vi "CreateScanPattern_LS1.vi"(8 "Error in":errorcluster, 11 "VarParam":string caption="Paramètre de balayage:") -> (0 "Error out":errorcluster, 1 "ModèleSauv":i32, 2 "SavedOK":bool, 3 "Modèles out":string[](array[string]))   [LabVIEW 2010]
doc: "Ce Vi sert à la création de modèles de balayages. À partir des positions de départ, de fin et du pas du balayage, il crée une liste de position qui constitue le modèle. Le VI permet ensuite la sauvegarde des nouveaux modèles et la gestion des modèles existant."
uses:
  <vilib>/Utility/error.llb/DialogType.ctl
  <vilib>/Utility/config.llb/NI_LVConfig.lvlib
panel:
  out "VarParamOut":string caption="Paramètre de balayage:"
  in  "InclFin":bool=TRUE caption="Inclure la \nposition finale"
  in  "Positions":dbl[](array[numeric])=[-100.0, -90.0, -80.0, -70.0, -60.0, -50.0, -40.0, -30.0, -20.0, -10.0, 0.0, 10.0, 20.0, 30.0, 40.0, 50.0, 60.0, 70.0, 80.0, 90.0, 100.0, 110.0, 120.0, 130.0, 140.0, 150.0, 160.0, 170.0, 180.0, 190.0, 200.0, 210.0, 220.0, 230.0, 240.0, 250.0, 260.0, 270.0, 280.0, 290.0, 300.0, 310.0, 320.0, 330.0, 340.0, 350.0, 360.0, 370.0, 380.0, 390.0, 400.0, 410.0, 420.0, 430.0, 440.0, 450.0, 460.0, 470.0, 480.0, 490.0, 500.0, 510.0, 520.0, 530.0, 540.0, 550.0, 560.0, 570.0, 580.0, 590.0, 600.0, 610.0, 620.0, 630.0, 640.0, 650.0, 660.0, 670.0, 680.0, 690.0, 700.0, 710.0, 720.0, 730.0, 740.0, 750.0, 760.0, 770.0, 780.0, 790.0, 800.0, 810.0, 820.0, 830.0, 840.0, 850.0, 860.0, 870.0, 880.0, 890.0, 900.0, 910.0, 920.0, 930.0, 940.0, 950.0, 960.0, 970.0, 980.0, 990.0, 1000.0] min=-2.0 max=770.0 step=0.01 format="%.2f"
  in  "OK":bool
  in  "Save":bool
  in  "Ajouter":bool
  in  "Effacer":bool
  in  "Fin":dbl=770.0 format="%.2f"
  in  "Pas":dbl=0.1 format="%.2f"
  in  "Départ":dbl=770.0 format="%.2f"
  in  "Nom du modèle":string
  in  "Modèles":i32(listbox) caption="Modèles de Balayage"
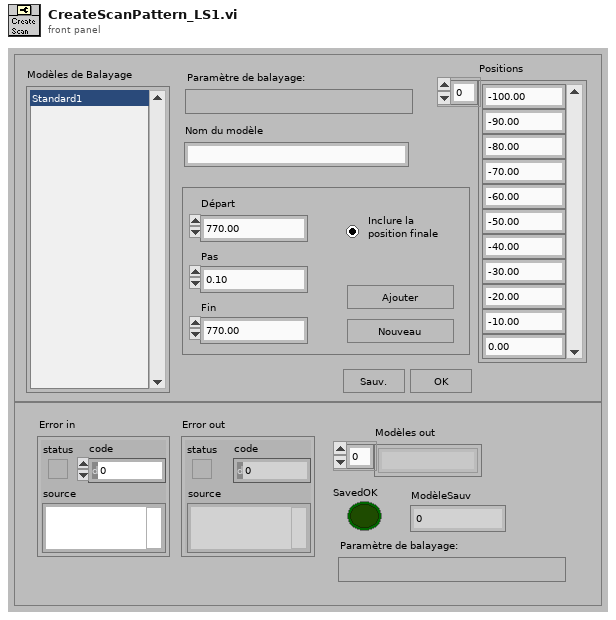
[diagram p1: front panel]
types:
  T1 = typedef "DialogType.ctl" = u16
  T2 = typedef "NI_LVConfig.lvlib/Config Data RefNum.ctl" = refnum<k1>
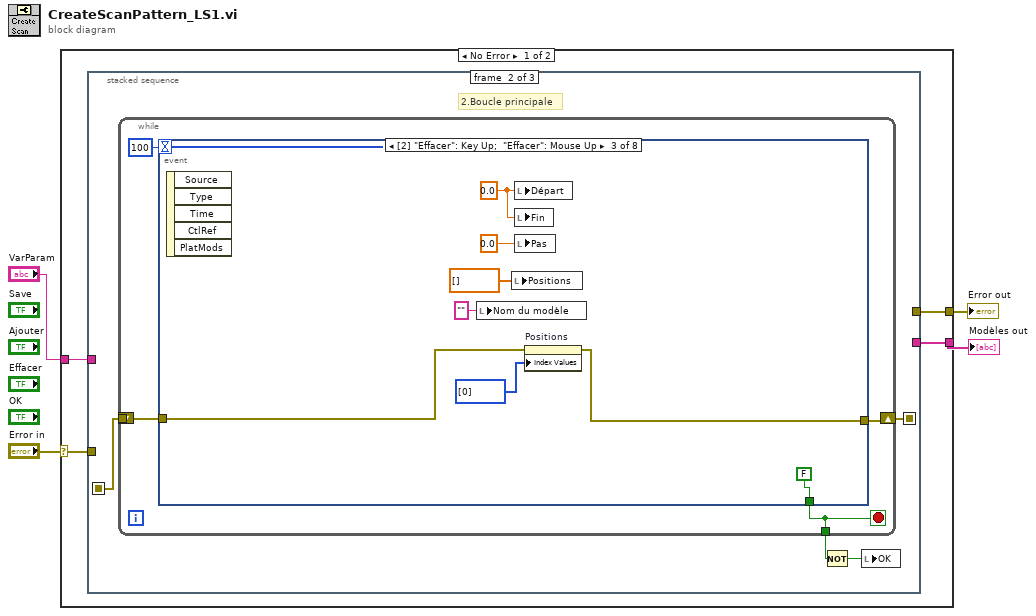
[diagram p0: block diagram]
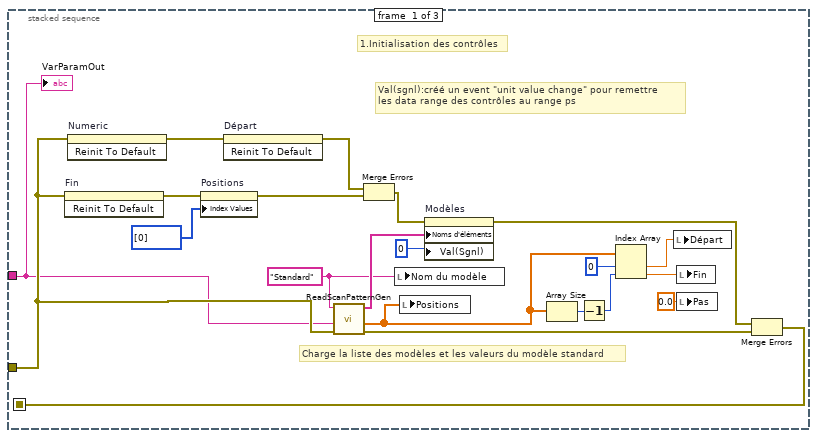
[diagram p2: hidden frame]
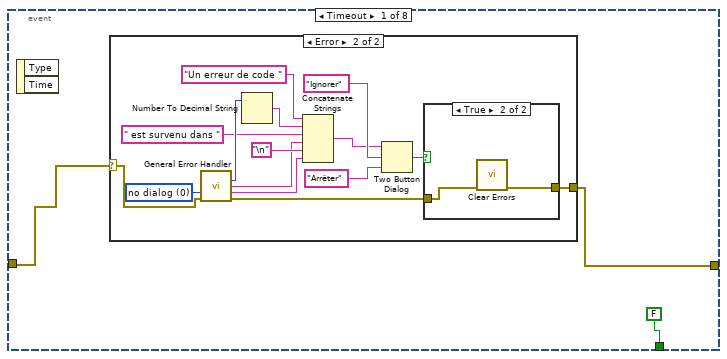
[diagram p3: hidden frame]
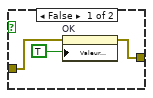
[diagram p5: hidden frame]
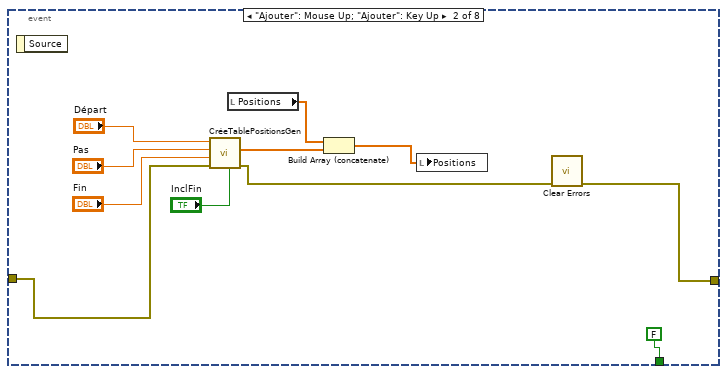
[diagram p6: hidden frame]
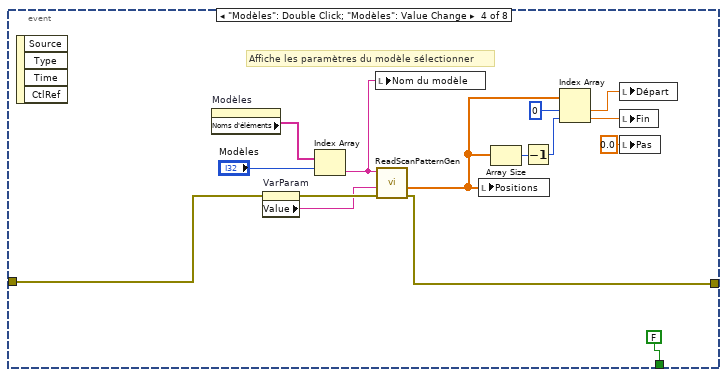
[diagram p7: hidden frame]
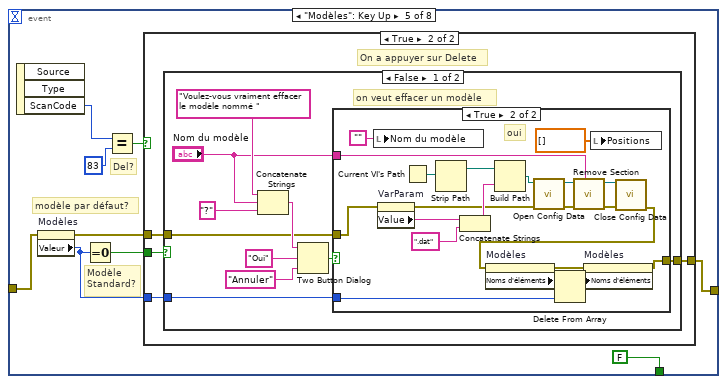
[diagram p8: hidden frame]
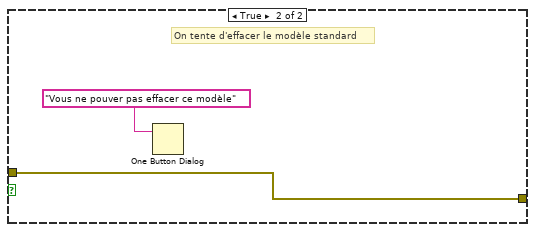
[diagram p11: hidden frame]
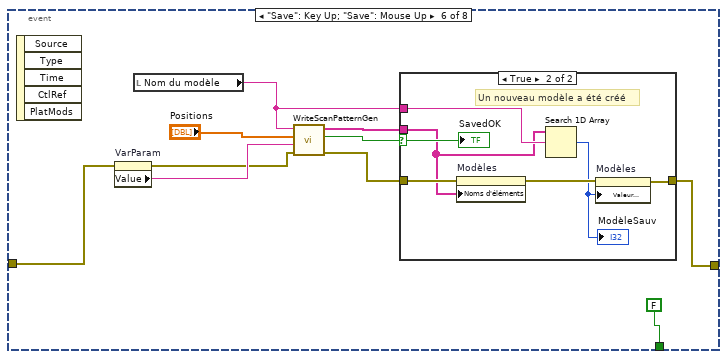
[diagram p12: hidden frame]
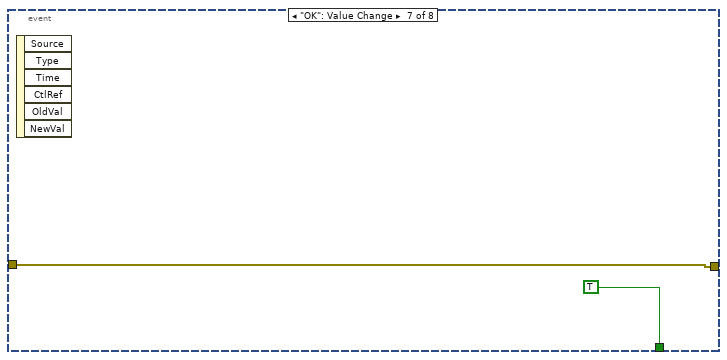
[diagram p14: hidden frame]
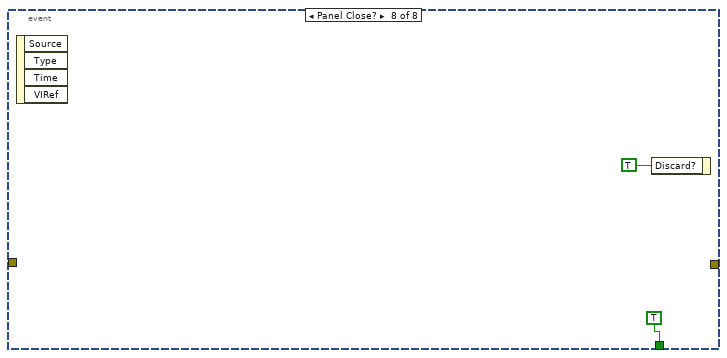
[diagram p15: hidden frame]
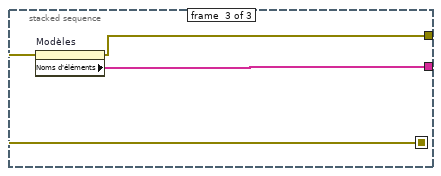
[diagram p16: hidden frame]
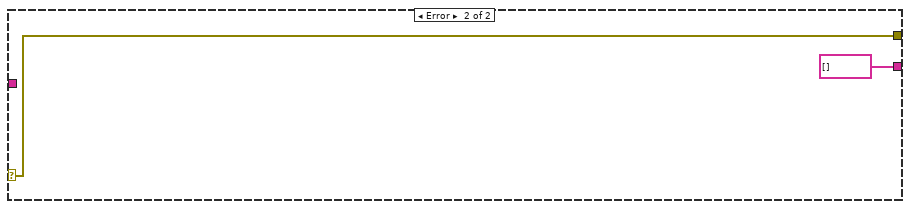
[diagram p17: hidden frame]
diagram:
  n1 = case shown="No Error" "Error in" {
    selector: "Error in" -> [w8 w170]
    tunnel: [w6 w170] -> w4
    tunnel: [w7 string[] [] ("Item Names")] -> w2
    tunnel: "VarParam" -> [w5 _]
    frame No Error {
      n2 = stacked-sequence {
        seq-local: [w27 _ _] -> [_ w33 _]
        seq-local: [_ w32 _] -> [_ _ w167]
        tunnel: w8 -> [w10 _ _]
        tunnel: [_ _ w168] -> w7
        tunnel: [_ _ w166] -> w6
        tunnel: w5 -> [w9 _ _]
        frame #0 {
          w23 = "Standard" ("Modèle")
          # "Val(sgnl):créé un event \"unit value change\" pour remettre \nles data range des contrôles au range ps"
          # "Charge la liste des modèles et les valeurs du modèle standard"
          # "1.Initialisation des contrôles"
          n3 = invoke on="Fin" class="Digital (strict)" method="Reinit To Default"(error in=w10) -> (error out=w13:errorcluster)  [unwired: 2 in, 2 out]
          n4 = invoke on="Numeric" class="DigNum (strict)" method="Reinit To Default"(error in=w10) -> (error out=w26:errorcluster)  [unwired: 2 in, 2 out]
          n5 = property on="Positions" class="Arr (strict)"(error in=w13, "Index Values"=u32[] [0] ("Valeurs d'indice")) -> (error out=w12:errorcluster)  [unwired: 1 in, 1 out]
          n6 = invoke on="Départ" class="Digital (strict)" method="Reinit To Default"(error in=w26) -> (error out=w25:errorcluster)  [unwired: 2 in, 2 out]
          n7 = call <userlib>:"ReadScanPatternGen.vi"("Error in"=w10, "VarParam"=w9, "Modèle"=w23) -> ("Error out"=w21:errorcluster, "Positions"=w16:dbl[], "Modèles"=w24:string[])  [unwired: 2 in]
          n8 = Merge Errors(w25, w12) -> (w29:errorcluster)
          n9 = local write "Nom du modèle"(w23) -> ()
          n10 = local write "Positions"(w16) -> ()
          n11 = property on="Modèles" class="LstBox (strict)"(error in=w29, "Noms d'éléments"=w24, "Val(Sgnl)"=0 ("Modèles")) -> (error out=w28:errorcluster)  [unwired: 1 in, 1 out]
          n12 = Array Size(array=w16) -> (size(s)=w18:i32)
          n13 = Decrement(x=w18) -> (x-1=w19:i32)
          n14 = Index Array(array=w16, index #1=0 ("index"), index #2=w19) -> (element #1=w20:dbl, element #2=w15:dbl)
          n15 = local write "Départ"(w20) -> ()
          n16 = local write "Fin"(w15) -> ()
          n17 = local write "Pas"(0.0 ("Pas")) -> ()
          n18 = Merge Errors(w28, w21) -> (w27:errorcluster)
          "VarParamOut" <- w9
        }
        frame #1 {
          # "2.Boucle principale"
          n19 = while {
            shift-right: [w36] -> w32
            shift-left: w33 -> [w35]
            tunnel: w33 -> [_]
            tunnel: [w34] -> w31
            stop <- w34 stop-if-true
            n20 = event shown="[2] \"Effacer\": Key Up;  \"Effacer\": Mouse Up" {
              selector: _ -> [_ _ _ _ _ _ _ _]
              dyn-events: _ -> [_ _ _ _ _ _ _ _]
              timeout: 100 -> [_ _ _ _ _ _ _ _]
              tunnel: [FALSE ("status") FALSE ("status") FALSE ("status") FALSE ("status") FALSE ("status") FALSE ("status") TRUE TRUE ("status")] -> w34
              tunnel: [w39 w66 w73 w94 w98 w151 w162 _] -> w36
              tunnel: w35 -> [w38 w68 w74 w83 w100 w145 w162 _]
              event Timeout {
                n21 = event-data() -> ()  [unwired: 1 in, 2 out]
                n22 = case shown="Error" w38 {
                  selector: w38 -> [w41 w42]
                  tunnel: [w41 w43] -> w39
                  frame No Error {
                  }
                  frame Error {
                    w53 = T1 0 items=["no dialog", "OK message", "continue or stop message", "OK message + warnings", "continue/stop + warnings"] ("type of dialog (OK msg:1)")
                    n23 = call <vilib>:"General Error Handler.vi"("type of dialog (OK msg:1)"=w53, "error in (no error)"=w42) -> ("code out"=w49:i32, "source out"=w48:string, "message"=w46:string, "error out"=w44:errorcluster)  [unwired: 9 in, 1 out]
                    n24 = Number To Decimal String(number=w49) -> (decimal integer string=w50:string)  [unwired: 1 in]
                    n25 = Concatenate Strings("Un erreur de code " ("string"), w50, " est survenu dans " ("string"), w48, "\n", w46) -> (w45:string)
                    n26 = Two Button Dialog(message=w45, 1:"Arrêter" ("F button name (\"Cancel\")"), 2:"Ignorer" ("T button name (\"OK\")")) -> (T button?=w56:bool)
                    n27 = case shown="True" w56 {
                      tunnel: w44 -> [w58 w61]
                      tunnel: [w57 w60] -> w43
                      frame False {
                        n28 = property on="OK" class="Bool (strict)"(error in=w58, "Valeur (Signalisation)"=TRUE ("Value (Signaling)")) -> (error out=w57:errorcluster)  [unwired: 1 in, 1 out]
                      }
                      frame True {
                        n29 = call <vilib>:"Clear Errors.vi"("error in (no error)"=w61) -> ("error out"=w60:errorcluster)  [unwired: 6 in]
                      }
                    }
                  }
                }
              }
              event "Ajouter": Mouse Up; "Ajouter": Key Up {
                n30 = event-data() -> ()  [unwired: 1 in, 1 out]
                n31 = call <userlib>:"CréeTablePositionsGen.vi"("IncFin (T)"="InclFin", "error in (no error)"=w68, "Fin"="Fin", "Increment"="Pas", "Debut"="Départ") -> ("error out"=w67:errorcluster, "Positions"=w64:dbl[])  [unwired: 4 in, 1 out]
                n32 = local read "Positions"() -> (w63:dbl[])
                n33 = Build Array (concatenate)(w63, w64) -> (w62:dbl[])
                n34 = local write "Positions"(w62) -> ()
                n35 = call <vilib>:"Clear Errors.vi"("error in (no error)"=w67) -> ("error out"=w66:errorcluster)  [unwired: 6 in]
              }
              event "Effacer": Key Up; "Effacer": Mouse Up {
                w78 = 0.0 ("Départ")
                n36 = event-data() -> ()  [unwired: 1 in, 5 out]
                n37 = local write "Nom du modèle"("" ("Nom du modèle")) -> ()
                n38 = local write "Positions"(dbl[] [] ("Positions")) -> ()
                n39 = local write "Départ"(w78) -> ()
                n40 = local write "Fin"(w78) -> ()
                n41 = local write "Pas"(0.0 ("Pas")) -> ()
                n42 = property on="Positions" class="Arr (strict)"(error in=w74, "Index Values"=u32[] [0] ("Valeurs d'indice")) -> (error out=w73:errorcluster)  [unwired: 1 in, 1 out]
              }
              event "Modèles": Double Click; "Modèles": Value Change {
                # "Affiche les paramètres du modèle sélectionner"
                n43 = event-data() -> ()  [unwired: 1 in, 4 out]
                n44 = property on="Modèles" class="LstBox (strict)"() -> ("Noms d'éléments"=w92:string[])  [unwired: 2 in, 2 out]
                n45 = property on="VarParam" class="Str"(error in=w83) -> (error out=w82:errorcluster, "Value"=w81:string)  [unwired: 1 in, 1 out]
                n46 = Index Array(array=w92, index="Modèles") -> (element=w95:string)
                n47 = local write "Nom du modèle"(w95) -> ()
                n48 = call <userlib>:"ReadScanPatternGen.vi"("Error in"=w82, "VarParam"=w81, "Modèle"=w95) -> ("Error out"=w94:errorcluster, "Positions"=w87:dbl[])  [unwired: 2 in, 1 out]
                n49 = local write "Positions"(w87) -> ()
                n50 = Array Size(array=w87) -> (size(s)=w89:i32)
                n51 = Decrement(x=w89) -> (x-1=w90:i32)
                n52 = Index Array(array=w87, index #1=0 ("index"), index #2=w90) -> (element #1=w91:dbl, element #2=w86:dbl)
                n53 = local write "Départ"(w91) -> ()
                n54 = local write "Fin"(w86) -> ()
                n55 = local write "Pas"(0.0 ("Pas")) -> ()
              }
              event "Modèles": Key Up {
                # "Modèle\nStandard?"
                # "Del?"
                # "modèle par défaut?"
                n56 = event-data() -> ("ScanCode"=w104:i16)  [unwired: 1 in, 2 out]
                n57 = property on="Modèles" class="LstBox (strict)"(error in=w100) -> (error out=w99:errorcluster, "Valeur"=w101:i32)  [unwired: 1 in, 1 out]
                n58 = Equal To 0?(x=w101) -> (x = 0?=w102:bool)
                n59 = Equal?(x=w104, y=i16 83) -> (x = y?=w103:bool)
                n60 = case shown="True" w103 {
                  tunnel: w102 -> [_ w109]
                  tunnel: w101 -> [_ w108]
                  tunnel: w99 -> [w105 w107]
                  tunnel: [w105 w106] -> w98
                  frame False {
                  }
                  frame True {
                    # "On a appuyer sur Delete"
                    n61 = case shown="False" w109 {
                      tunnel: w108 -> [w113 _]
                      tunnel: w107 -> [w112 w142]
                      tunnel: [w111 w142] -> w106
                      frame False {
                        # "on veut effacer un modèle"
                        n62 = Concatenate Strings("Voulez-vous vraiment effacer le modèle nommé " ("string"), "Nom du modèle", "?" ("string")) -> (w117:string)
                        n63 = Two Button Dialog(message=w117, 1:"Annuler" ("T button name (\"OK\")"), 2:"Oui" ("T button name (\"OK\")")) -> (T button?=w114:bool)
                        n64 = case shown="True" w114 {
                          tunnel: w113 -> [_ w129]
                          tunnel: w112 -> [w120 w123]
                          tunnel: [w120 w130] -> w111
                          tunnel: "Nom du modèle" -> [_ w134]
                          frame False {
                            # "non : effaçage annuler"
                          }
                          frame True {
                            # "oui"
                            n65 = local write "Nom du modèle"("") -> ()
                            n66 = property on="VarParam" class="Str"(error in=w123) -> (error out=w122:errorcluster, "Value"=w121:string)  [unwired: 1 in, 1 out]
                            n67 = Current VI's Path() -> (path=w139:path)
                            n68 = Strip Path(path=w139) -> (stripped path=w140:path)  [unwired: 1 out]
                            n69 = Concatenate Strings(w121, ".dat" ("chaîne")) -> (w125:string)
                            n70 = Build Path(base path=w140, name or relative path=w125) -> (appended path=w141:path)
                            n71 = call <vilib>:"Open Config Data.vi"("error in (no error)"=w122, "configuration file path"=w141) -> ("error out"=w138:errorcluster, "refnum"=w137:T2)  [unwired: 7 in, 1 out]
                            n72 = call <vilib>:"Remove Section.vi"("section"=w134, "error in (no error)"=w138, "refnum"=w137) -> ("error out"=w135:errorcluster, "refnum out"=w136:T2)  [unwired: 6 in, 1 out]
                            n73 = local write "Positions"(dbl[] [] ("Positions")) -> ()
                            n74 = call <vilib>:"Close Config Data.vi"("error in (no error)"=w135, "refnum"=w136) -> ("error out"=w131:errorcluster)  [unwired: 8 in, 1 out]
                            n75 = property on="Modèles" class="LstBox (strict)"(error in=w131) -> (error out=w132:errorcluster, "Noms d'éléments"=w133:string[])  [unwired: 1 in, 1 out]
                            n76 = Delete From Array(array=w133, index=w129) -> (array with subset deleted=w128:string[])  [unwired: 1 in, 1 out]
                            n77 = property on="Modèles" class="LstBox (strict)"(error in=w132, "Noms d'éléments"=w128) -> (error out=w130:errorcluster)  [unwired: 1 in, 1 out]
                          }
                        }
                      }
                      frame True {
                        # "On tente d'effacer le modèle standard"
                        n78 = One Button Dialog(message="Vous ne pouver pas effacer ce modèle") -> ()  [unwired: 1 in, 1 out]
                      }
                    }
                  }
                }
              }
              event "Save": Key Up; "Save": Mouse Up {
                n79 = event-data() -> ()  [unwired: 1 in, 5 out]
                n80 = property on="VarParam" class="Str"(error in=w145) -> (error out=w144:errorcluster, "Value"=w146:string)  [unwired: 1 in, 1 out]
                n81 = local read "Nom du modèle"() -> (w148:string)
                n82 = call <userlib>:"WriteScanPatternGen.vi"("Error in"=w144, "VarParam"=w146, "Positions"="Positions", "Modèle"=w148) -> ("Error out"=w152:errorcluster, "SavedOK"=w153:bool, "Modèles"=w150:string[])  [unwired: 4 in]
                n83 = case shown="True" w153 {
                  selector: w153 -> [_ w160]
                  tunnel: [w154 w158] -> w151
                  tunnel: w152 -> [w154 w161]
                  tunnel: w150 -> [_ w156]
                  tunnel: w148 -> [_ w157]
                  frame False {
                    # "La création n'a pas eu lieu"
                  }
                  frame True {
                    # "Un nouveau modèle a été créé"
                    n84 = property on="Modèles" class="LstBox (strict)"(error in=w161, "Noms d'éléments"=w156) -> (error out=w159:errorcluster)  [unwired: 1 in, 1 out]
                    n85 = Search 1D Array(1D array=w156, element=w157) -> (index of element=w155:i32)  [unwired: 1 in]
                    "ModèleSauv" <- w155
                    n86 = property on="Modèles" class="LstBox (strict)"(error in=w159, "Valeur (Signalisation)"=w155) -> (error out=w158:errorcluster)  [unwired: 1 in, 1 out]
                    "SavedOK" <- w160
                  }
                }
              }
              event "OK": Value Change {
                n87 = event-data() -> ()  [unwired: 1 in, 6 out]
              }
              event Panel Close? {
                n88 = event-data() -> ()  [unwired: 1 in, 4 out]
                n89 = event-data("Discard?"=TRUE) -> ()  [unwired: 1 in, 1 out]
              }
            }
          }
          n90 = Not(x=w31) -> (.not. x?=w30:bool)
          n91 = local write "OK"(w30) -> ()
        }
        frame #2 {
          n92 = property on="Modèles" class="LstBox (strict)"(error in=w167) -> (error out=w166:errorcluster, "Noms d'éléments"=w168:string[])  [unwired: 1 in, 1 out]
        }
      }
    }
    frame Error {
    }
  }
  "Error out" <- w4
  "Modèles out" <- w2
